vi "DIAdem Opened Check.vi"(0 "error in (no error)":errorcluster) -> (1 "DIAdem Window Refnum":T1, 2 "DIAdem Window Handle":i32, 3 "DIAdem Opened":bool, 4 "error out":errorcluster)   [LabVIEW 2020]
doc: "This VI checks whether DIAdem is opened."
uses:
  <vilib>/ExportToExcel/Window Refnum.ctl
  user32.dll
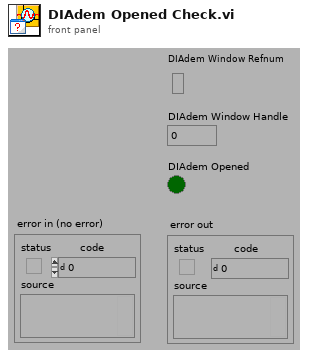
[diagram p1: front panel]
types:
  T1 = typedef "Window Refnum.ctl" = refnum<k1>
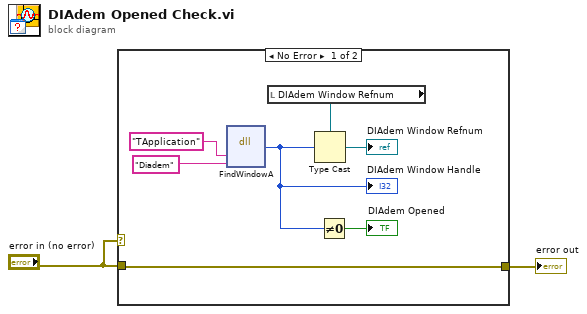
[diagram p0: block diagram]
diagram:
  n1 = case shown="No Error" "error in (no error)" {
    tunnel: "error in (no error)" -> [w3 w10]
    tunnel: [w3 w10] -> w2
    frame No Error {
      n2 = dll-call lib="user32.dll" fn="FindWindowA"("ClassName"="TApplication", "WindowName"="Diadem") -> (w7:u32)  [unwired: 5 in, 2 out]
      "DIAdem Window Handle" <- w7
      n3 = local read "DIAdem Window Refnum"() -> (w6:T1)
      n4 = Type Cast(type=w6, x=w7) -> (*(type *) &x=→"DIAdem Window Refnum":T1)
      n5 = Not Equal To 0?(x=w7) -> (x != 0?=→"DIAdem Opened":bool)
    }
    frame Error {
    }
  }
  "error out" <- w2
